vi "NI VeriStand - Close Alarm.vi"(8 "error in (no error)":errorcluster, 11 "Alarm":T1) -> (0 "error out":errorcluster)   [LabVIEW 2020, in "NI_VS Alarm ExecutionAPI.lvlib"]
doc: "Closes an open reference to an alarm. Use this VI to close each alarm reference that you open with the Open Alarm VI."
uses:
  <vilib>/NI VeriStand/Execution/Alarm/NI_VS Alarm ExecutionAPI.lvlib
  <vilib>/NI VeriStand/Execution/Alarm/AlarmAPI.ctl
  NationalInstruments.VeriStand.ClientAPI
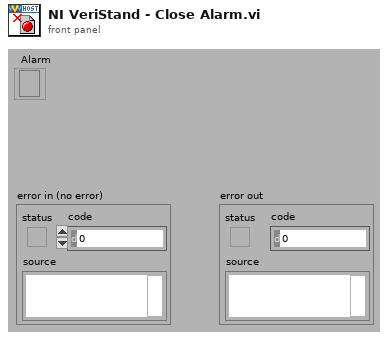
[diagram p1: front panel]
types:
  T1 = typedef "NI_VS Alarm ExecutionAPI.lvlib/AlarmAPI.ctl" = refnum<k24>
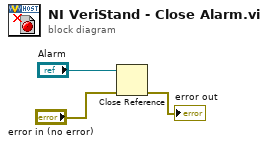
[diagram p0: block diagram]
diagram:
  n1 = Close Reference(reference="Alarm", error in (no error)="error in (no error)") -> (error out=→"error out":errorcluster)
